vi "kalibracja_gensig.vi"(4 "NI device/channel":tag="1/ai0", 5 "Averages":u32(slide)=128 scale=0.0..1024.0 scale format="%.2f", 6 "error in":errorcluster, 7 "Sampling frequency [Hz]":dbl(slide)=100000.0 step=10000.0 scale=50000.0..150000.0) -> (0 "error out":errorcluster, 1 "mean":dbl, 2 "Array":dbl[](array[numeric]), 3 "Spectrum Plot":cluster{dbl, "df":dbl, "Spectrum out":dbl[]}(graph))   [LabVIEW 2013]
uses:
  <vilib>/Analysis/1siggen.llb/Ramp Pattern by Samples.vi
  <vilib>/DAQmx/read.llb/DAQmx Read (Analog 1D DBL 1Chan NSamp).vi
  <vilib>/DAQmx/create/channels.llb/DAQmx Create Channel (AI-Voltage-Basic).vi
  <vilib>/DAQmx/configure/timing.llb/DAQmx Timing (Sample Clock).vi
  <vilib>/DAQmx/miscellaneous.llb/DAQmx Fill In Error Info.vi
  <vilib>/Analysis/NI_AALPro.lvlib
  <vilib>/Analysis/NI_AALBase.lvlib
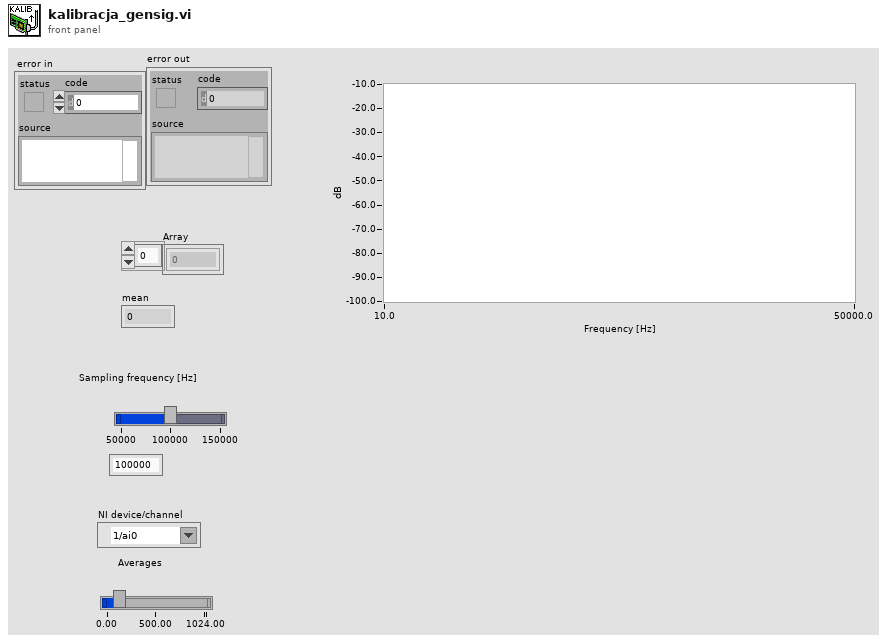
[diagram p1: front panel]
types:
  T1 = enum32{"Vrms", "Vpk", "Vrms^2", "Vpk^2", "Vrms/rtHz", "Vpk/rtHz", "Vrms^2/Hz", "Vpk^2/Hz"}
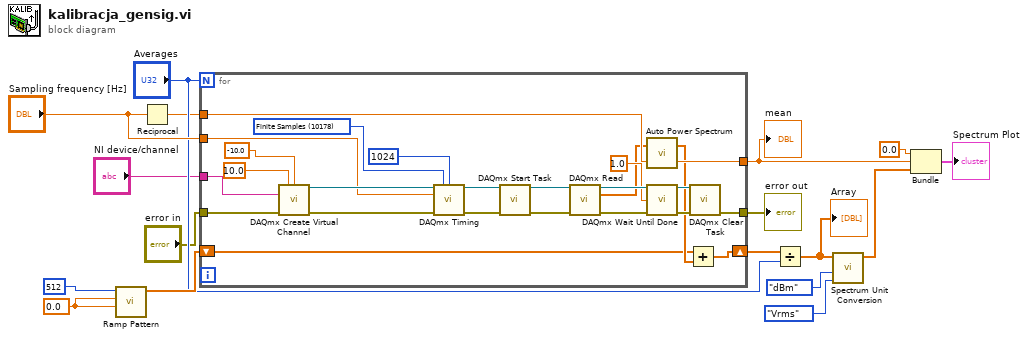
[diagram p0: block diagram]
diagram:
  w12 = 0.0
  n1 = call-poly <vilib>:"Ramp Pattern.vi"("start"=w12, "end"=w12, "samples"=i16 512) -> ("Ramp Pattern"=w15:dbl[])  [unwired: 7 in, 1 out]
  n2 = Reciprocal(x="Sampling frequency [Hz]") -> (1/x=w9:dbl)
  n3 = for {
    N: "Averages" -> [_]
    tunnel: [w42] -> w1
    tunnel: "NI device/channel" -> [w41]
    tunnel: w9 -> [w40]
    tunnel: "Sampling frequency [Hz]" -> [w21]
    shift-right: [w23] -> w10
    shift-left: w15 -> [w24]
    tunnel: "error in" -> [w19]
    tunnel: [w18] -> w2
    w27 = 10178 items=["Finite Samples"=10178, "Continuous Samples"=10123, "Hardware Timed Single Point"=12522] ("sample mode")
    n4 = call-poly <vilib>:"DAQmx Create Virtual Channel.vi"("maximum value"=10.0, "minimum value"=-10.0, "physical channels"=w41, "error in"=w19) -> ("task out"=w32:refnum<k21>, "error out"=w30:errorcluster)  [unwired: 10 in]
    n5 = call-poly <vilib>:"DAQmx Timing.vi"("task/channels in"=w32, "sample mode"=w27, "samples per channel"=1024, "rate"=w21, "error in"=w30) -> ("task out"=w31:refnum<k21>, "error out"=w29:errorcluster)  [unwired: 9 in]
    n6 = call <vilib>:"DAQmx Start Task.vi"("task/channels in"=w31, "error in"=w29) -> ("task out"=w37:refnum<k21>, "error out"=w28:errorcluster)  [unwired: 12 in]
    n7 = call-poly <vilib>:"DAQmx Read.vi"("task/channels in"=w37, "error in"=w28) -> ("task out"=w36:refnum<k21>, "data"=w20:dbl[], "error out"=w34:errorcluster)  [unwired: 11 in]
    n8 = call <vilib>:"Auto Power Spectrum.vi"("dt"=w40, "Signal (V)"=w20) -> ("df"=w42:dbl, "Power Spectrum (V^2 rms)"=w25:dbl[])
    n9 = call <vilib>:"DAQmx Wait Until Done.vi"("task/channels in"=w36, "timeout (sec)"=1.0, "error in"=w34) -> ("task out"=w35:refnum<k21>, "error out"=w33:errorcluster)  [unwired: 11 in]
    n10 = Add(x=w24, y=w25) -> (x+y=w23:dbl[])
    n11 = call <vilib>:"DAQmx Clear Task.vi"("task in"=w35, "error in"=w33) -> ("error out"=w18:errorcluster)  [unwired: 13 in]
  }
  "mean" <- w1
  "error out" <- w2
  n12 = Divide(x=w10, y="Averages") -> (x/y=w17:dbl[])
  "Array" <- w17
  n13 = call <vilib>:"Spectrum Unit Conversion.vi"("display unit"=T1."Vrms", "log/linear"=enum16{"Linear", "dB", "dBm"}."dBm" ("Log/Linear"), "Spectrum in"=w17) -> ("Spectrum out"=w4:dbl[])  [unwired: 7 in, 1 out]
  n14 = Bundle(0.0, "df"=w1, "Spectrum out"=w4) -> (→"Spectrum Plot":cluster{dbl, "df":dbl, "Spectrum out":dbl[]})  [unwired: 1 in]
